vi "Generic Instrument Finder.vi"() -> (1 "All Instruments found":T1(array[cluster]))   [LabVIEW 2013, in "Generic Instrument.lvlib" / "Generic Instrument.lvclass"]
uses:
  Generic Instrument.lvclass
  <vilib>/Instr/_visa.llb/VISA Open Access Mode.ctl
panel:
  out "error out":errorcluster
  in  "error in (no error)":errorcluster
  out "Boolean":bool
  out "read buffer":string
  out "find list":string[](array[string])
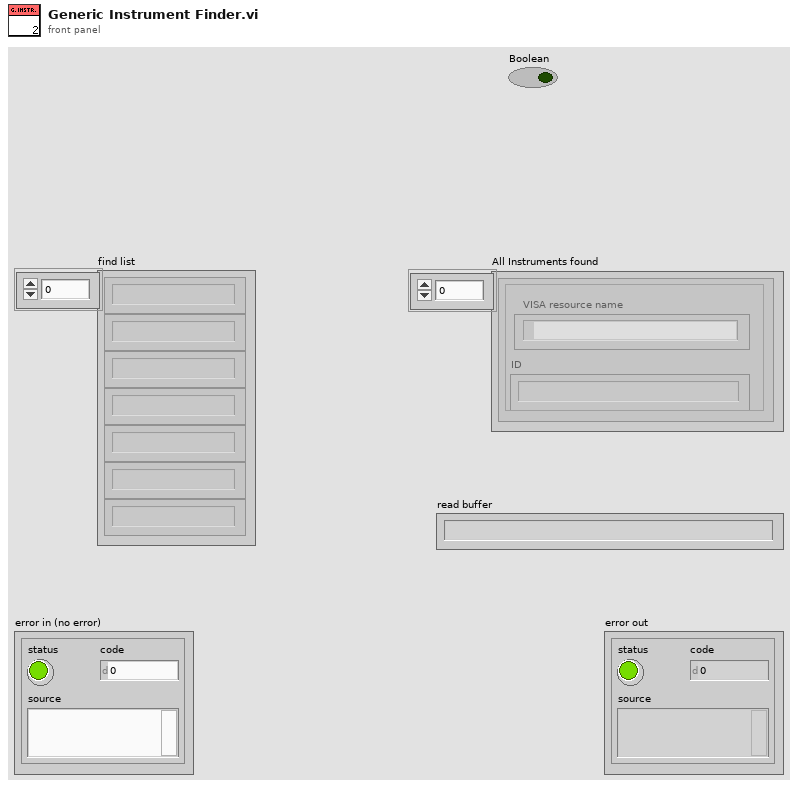
[diagram p1: front panel]
types:
  T1 = cluster{"VISA resource name":refnum<visa-resource-name>, "ID":string}[]
  T2 = typedef "VISA Open Access Mode.ctl" = u32
  T3 = cluster{"VISA resource name":refnum<visa-resource-name>, "read buffer":string}
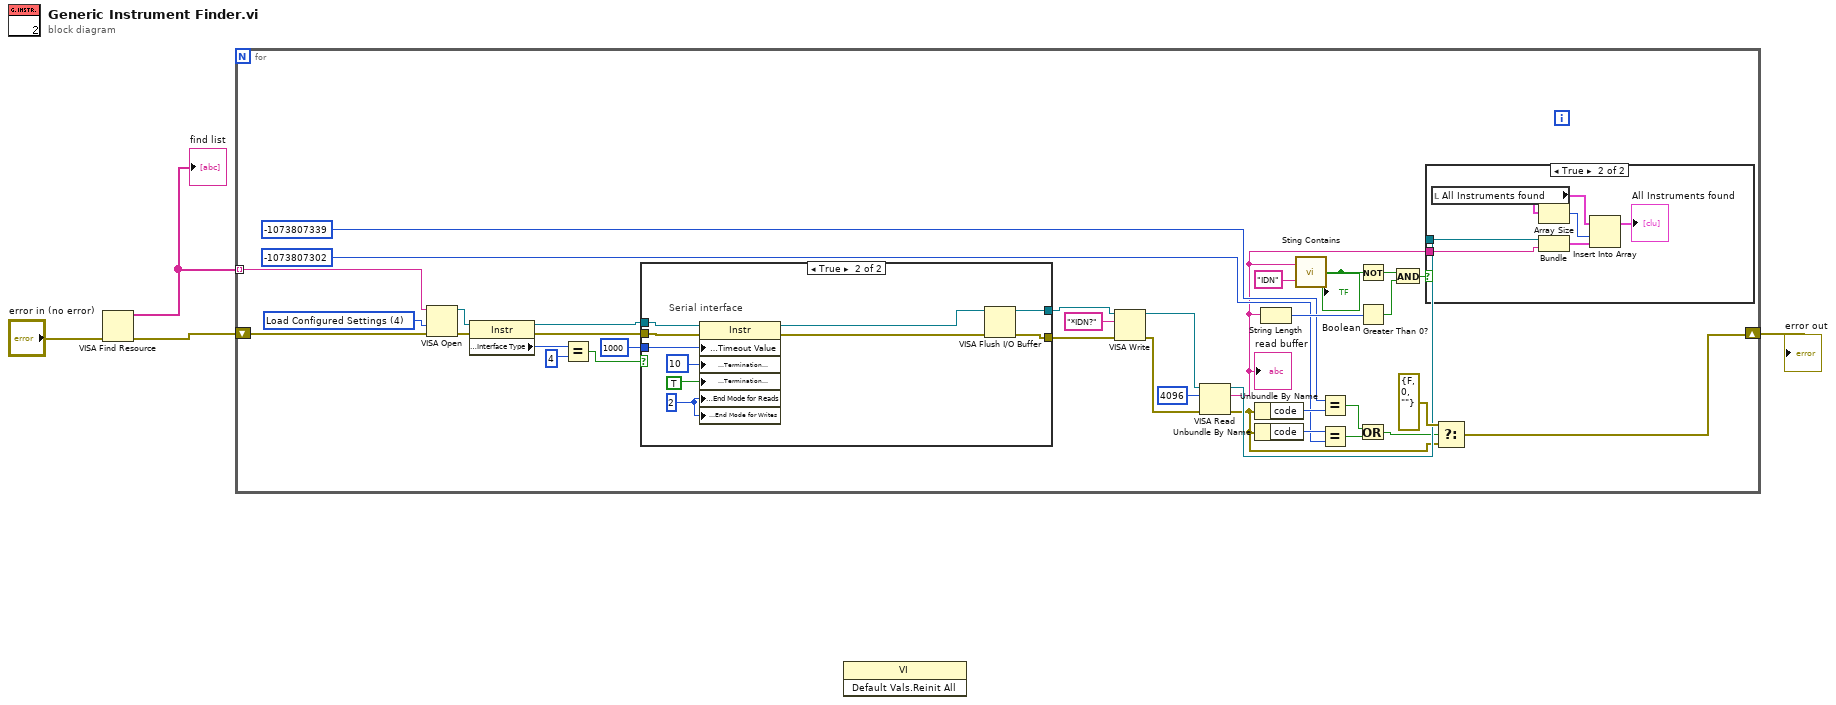
[diagram p0: block diagram]
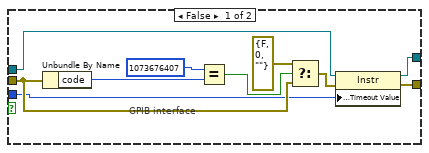
[diagram p3: hidden frame]
diagram:
  n1 = VISA Find Resource(8:"error in (no error)") -> (0:w3:errorcluster, 3:w4:string[])  [unwired: 2 in, 1 out]
  "find list" <- w4
  n2 = for {
    tunnel: w4 -> [w39] mode=indexing
    shift-right: [w22] -> w2
    shift-left: w3 -> [w37]
    w38 = T2 4 items=["VISA Defaults"=0, "Exclusive Lock"=1, "Load Configured Settings"=4] ("Access Mode")
    n3 = VISA Open(access mode=w38, error in (no error)=w37, VISA resource name=w39) -> (VISA resource name=w36:refnum<visa-resource-name>, error out=w35:errorcluster)  [unwired: 2 in]
    n4 = property class="Instr"(reference=w36, error in=w35) -> (reference out=w33:refnum<visa-resource-name>, error out=w34:errorcluster, "Interface Information:Interface Type"=w32:u16)
    n5 = Equal?(x=w32, y=u16 4) -> (x = y?=w30:bool)
    n6 = case shown="True" w30 {
      tunnel: [w55 w58] -> w26
      tunnel: [w54 w57] -> w17
      tunnel: w33 -> [w53 w62]
      tunnel: w34 -> [w49 w61]
      tunnel: u32 1000 ("Tmo Value") -> [w46 w56]
      frame False {
        # "GPIB interface"
        n7 = Unbundle By Name(w49) -> ("code"=w52:i32)
        n8 = Equal?(x=1073676407, y=w52) -> (x = y?=w50:bool)
        n9 = Select(t=errorcluster {"status"=FALSE, "code"=0, "source"=""}, s=w50, f=w49) -> (s? t:f=w47:errorcluster)
        n10 = property class="Instr"(reference=w53, error in=w47, "General Settings:Timeout Value"=w46) -> (reference out=w55:refnum<visa-resource-name>, error out=w54:errorcluster)
      }
      frame True {
        w63 = u16 2
        # "Serial interface"
        n11 = property class="Instr"(reference=w62, error in=w61, "General Settings:Timeout Value"=w56, "Message Based Settings:Termination Character"=u8 10, "Message Based Settings:Termination Character Enable"=TRUE, "Serial Settings:End Mode for Reads"=w63, "Serial Settings:End Mode for Writes"=w63) -> (reference out=w60:refnum<visa-resource-name>, error out=w59:errorcluster)
        n12 = VISA Flush I/O Buffer(VISA resource name=w60, error in (no error)=w59) -> (VISA resource name out=w58:refnum<visa-resource-name>, error out=w57:errorcluster)  [unwired: 1 in]
      }
    }
    n13 = VISA Write(VISA resource name=w26, write buffer="*IDN?", error in (no error)=w17) -> (VISA resource name out=w27:refnum<visa-resource-name>, error out=w18:errorcluster)  [unwired: 1 out]
    n14 = VISA Read(VISA resource name=w27, byte count=u32 4096, error in (no error)=w18) -> (VISA resource name out=w19:refnum<visa-resource-name>, read buffer=w10:string, error out=w16:errorcluster)  [unwired: 1 out]
    "read buffer" <- w10
    n15 = Unbundle By Name(w16) -> ("code"=w21:i32)
    n16 = Unbundle By Name(w16) -> ("code"=w15:i32)
    n17 = String Length(string=w10) -> (length=w25:i32)
    n18 = call "Sting Contains.vi"("Expression to evaluate"="IDN", "Input String"=w10) -> ("String Contains?"=w8:bool)
    "Boolean" <- w8
    n19 = Equal?(x=-1073807339 ("y"), y=w21) -> (x = y?=w12:bool)
    n20 = Equal?(x=w15, y=-1073807302) -> (x = y?=w13:bool)
    n21 = Not(x=w8) -> (.not. x?=w7:bool)
    n22 = Greater Than 0?(x=w25) -> (x > 0?=w6:bool)
    n23 = Or(x=w12, y=w13) -> (x .or. y?=w11:bool)
    n24 = And(x=w7, y=w6) -> (x .and. y?=w5:bool)
    n25 = case shown="True" w5 {
      tunnel: w19 -> [_ w44]
      tunnel: w10 -> [_ w43]
      frame False {
      }
      frame True {
        n26 = local read "All Instruments found"() -> (w41:T1)
        n27 = Array Size(array=w41) -> (size(s)=w40:i32)
        n28 = Bundle("VISA resource name"=w44, "read buffer"=w43) -> (w45:T3)  [unwired: 1 in]
        n29 = Insert Into Array(array=w41, index=w40, new element=w45) -> (→"All Instruments found":T1)
      }
    }
    n30 = Select(t=errorcluster {"status"=FALSE, "code"=0, "source"=""} ("error out"), s=w11, f=w16) -> (s? t:f=w22:errorcluster)
  }
  "error out" <- w2
  n31 = invoke class="VI" method="Default Vals.Reinit All"() -> ()  [unwired: 3 in, 3 out]
